vi "fpga_transmission_control_3V8.vi"() -> ()   [LabVIEW 2017]
uses:
  Control 1.ctl
  <vilib>/Platform/TimedLoop/XDataNode/timing_clust.ctl
  <vilib>/Platform/TimedLoop/XDataNode/nitl_modes.ctl
  <vilib>/Platform/TimedLoop/XDataNode/wakeup.ctl
  <vilib>/Instr/_visa.llb/VISA Configure Serial Port (Serial Instr).vi
  <vilib>/platform/TimedLoop/XDataNode/XDataNode.xnode
  <vilib>/Platform/TimedLoop/XDataNode/XDNodeRunTimeDep.lvlib
panel:
  out "Timer":dbl
  out "Output":bool
  out "outcome":u32
  out "currentType":string
  out "Time":dbl(slide) scale=0.0..100.0
  out "Progress":dbl(slide) scale=0.0..100.0
  in  "error in (no error)":errorcluster
  out "PWM":bool
  out "pattern":u32
  in  "Timeslot":bool
  out "type":string
  out "Kombi Chart":cluster{u16, i16}(graph)
  out "contingency":string
  in  "Array":T2(array[cluster]) {"duration" step=1}
  out "Timeslot":i32
  out "Sign":bool
  out "deleted portion":u8[](array[numeric])
  out "data":bool
  out "x-y":u16
  out "Error String":string
  out "error out":errorcluster
  out "Timing":u32
  out "Int_pixel":i16
  out "Pixel":u16(graph)
  out "AD_Value":i16
  in  "millisecond timer value 2":u32
  out "AD_Chart":i16(graph)
  in  "Path":path
  out "Read":bool
  in  "Stop Program":bool
  in  "Start":bool
  in  "VISA resource name":refnum<visa-resource-name>
  # "UR Elektronik Biologie\nTerminal V 3.8"
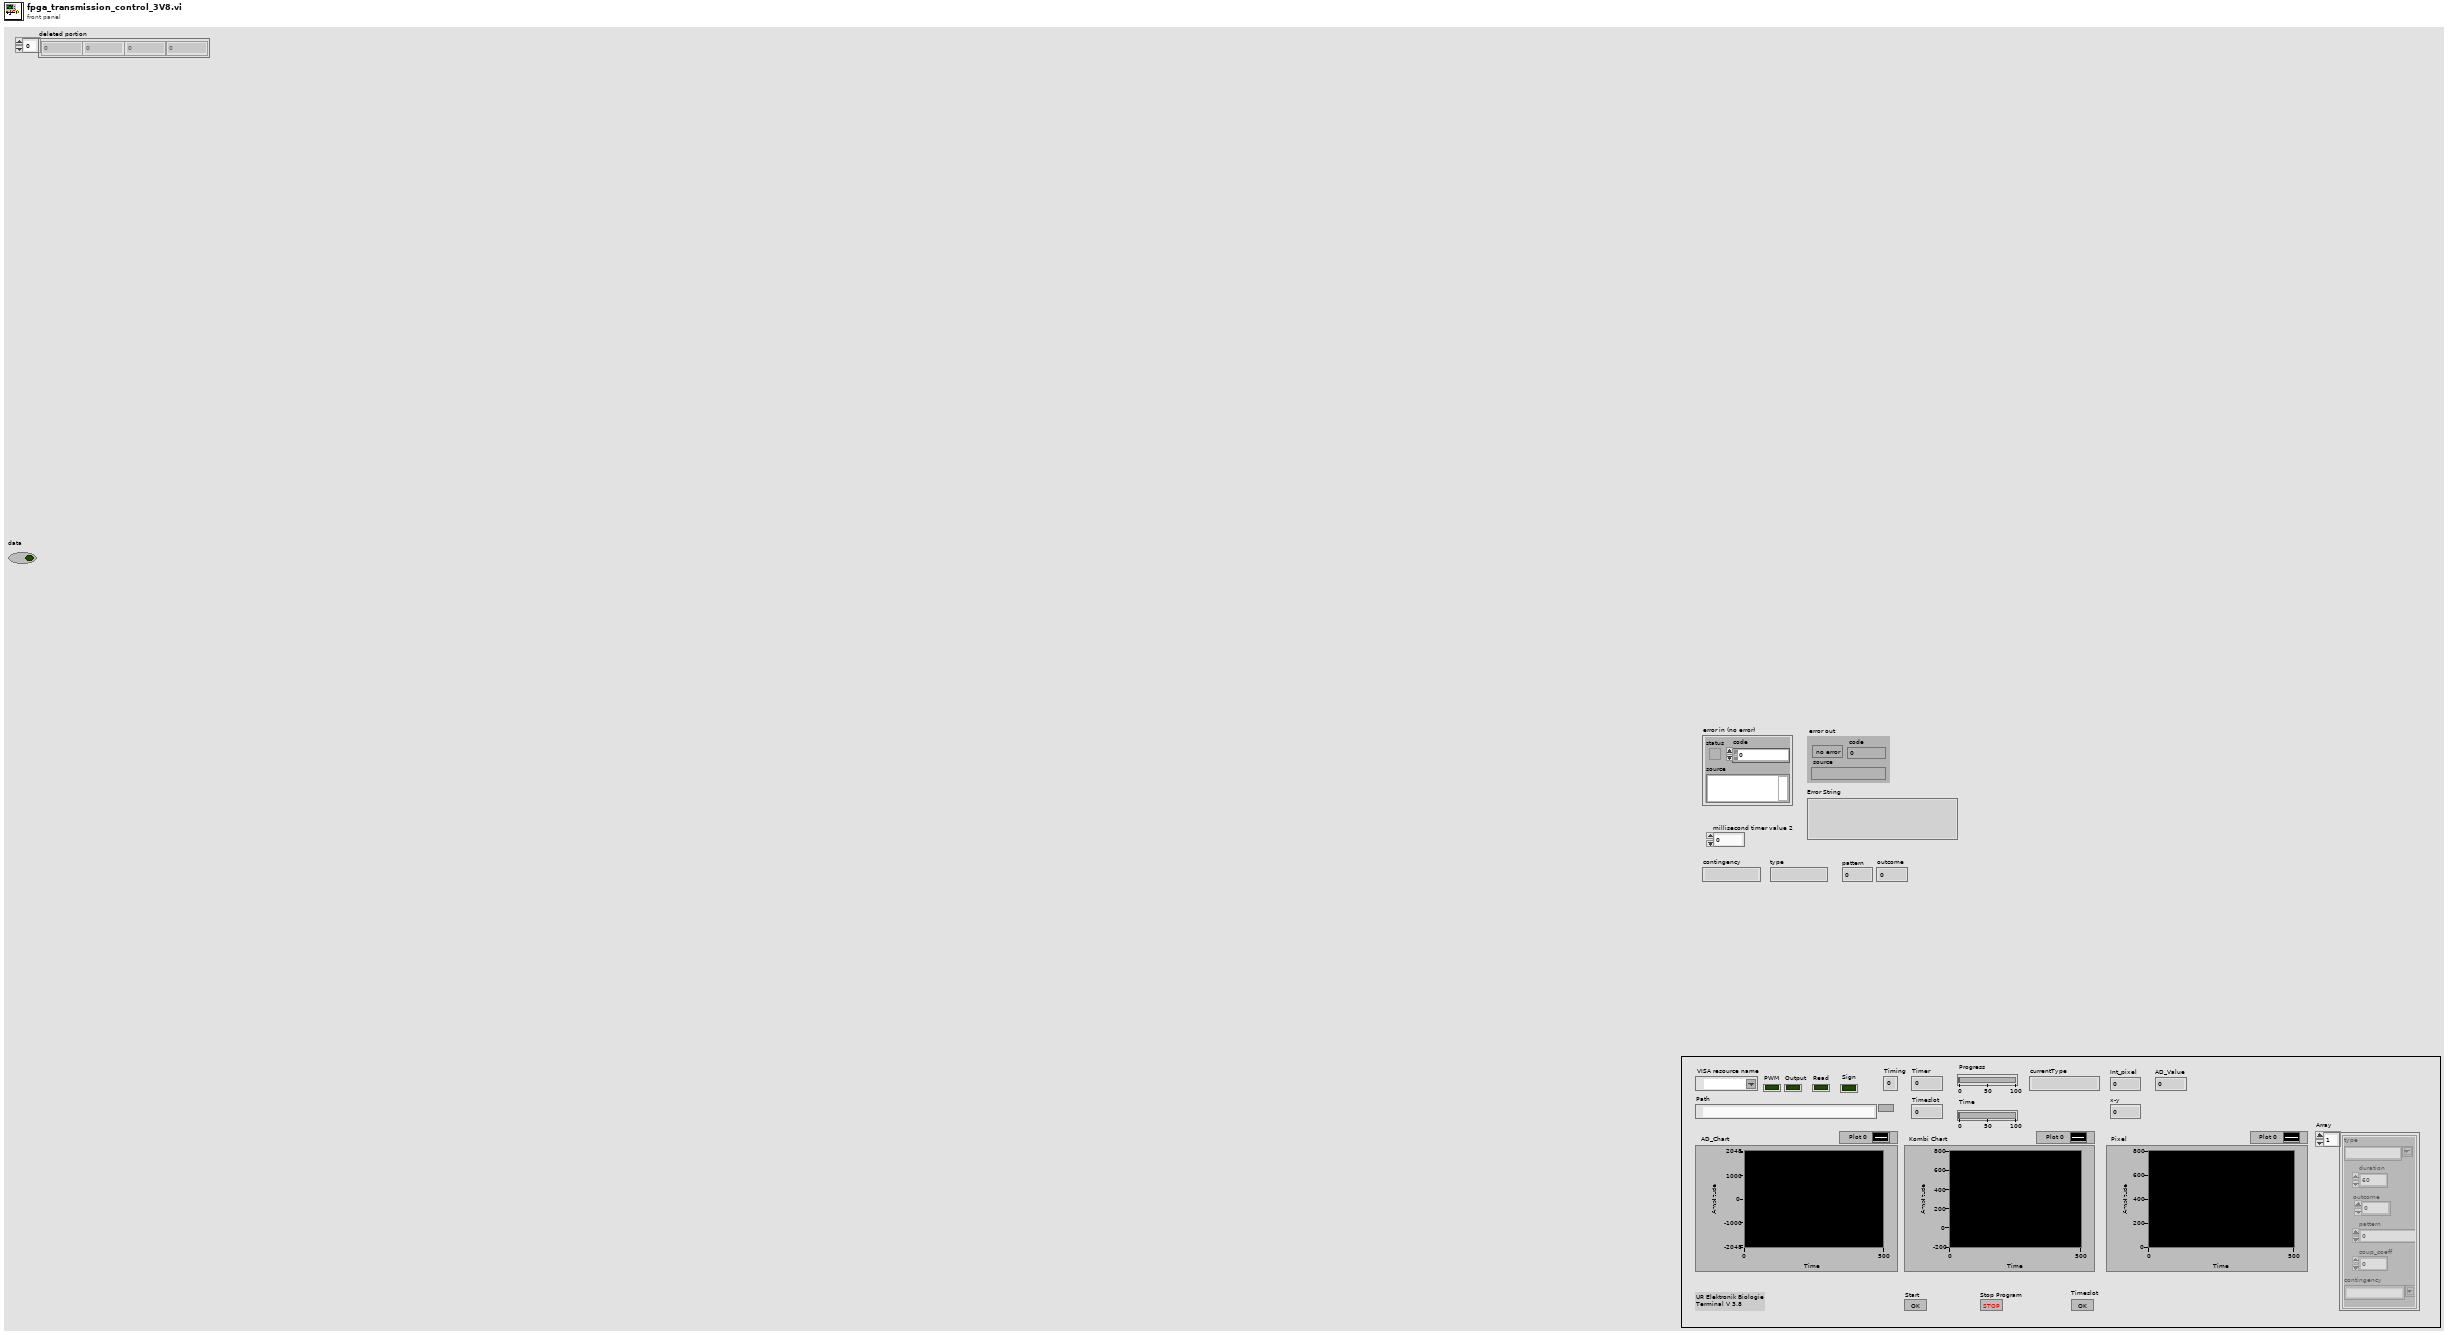
[diagram p1: front panel]
types:
  T1 = typedef "Control 1.ctl" = u32
  T2 = cluster{"type":string, "duration":T1, "outcome":u32, "pattern":u32, "coup_coeff":u32, "contingency":string}[]
  T3 = typedef "XDNodeRunTimeDep.lvlib/timing_clust.ctl" = cluster{"Expected End [f-1]":u64, "Actual End [f-1]":u64, "Finished Late? [f-1]":bool, "Expected End [i-1]":u64, "Actual End [i-1]":u64, "Finished Late? [i-1]":bool, "Expected Start [i]":u64, "Actual Start [i]":u64, "Expected Start [f]":u64, "Actual Start [f]":u64, "Source Name":string, "Structure Name":string, "Period":i64, "Deadline":i64, "Offset":i64, "Start":i64, "Priority":i32, "Timeout":i32, "Mode":T4, "Wakeup Reason":T5, "Error":errorcluster, "Source Type":string, "Secondary Source Type":string, "Global End Time":u64, "Global Start Time":u64, "Frame Duration":u64, "Iteration Duration":u64, "Assigned CPU":i32, "I/O Scan Engine Mode":u32}
  T4 = typedef "XDNodeRunTimeDep.lvlib/nitl_modes.ctl" = enum32{"No Change", "Process missed periods, maintain original phase", "Discard missed periods, maintain original phase", "Process missed periods, ignore original phase", "Discard missed periods, ignore original phase"}
  T5 = typedef "XDNodeRunTimeDep.lvlib/wakeup.ctl" = enum32{"Normal", "Aborted", "Asynchronous wakeup", "Timing source error", "Timed loop error", "Timeout"}
  T6 = cluster{"String":string, i32, i32, u32, u32, "String":string}[]
  T7 = enum16{"Idel", "State1", "State2", "State3", "State4"}
  T8 = enum16{"open", "replace", "create", "open or create", "replace or create", "replace or create with confirmation"}
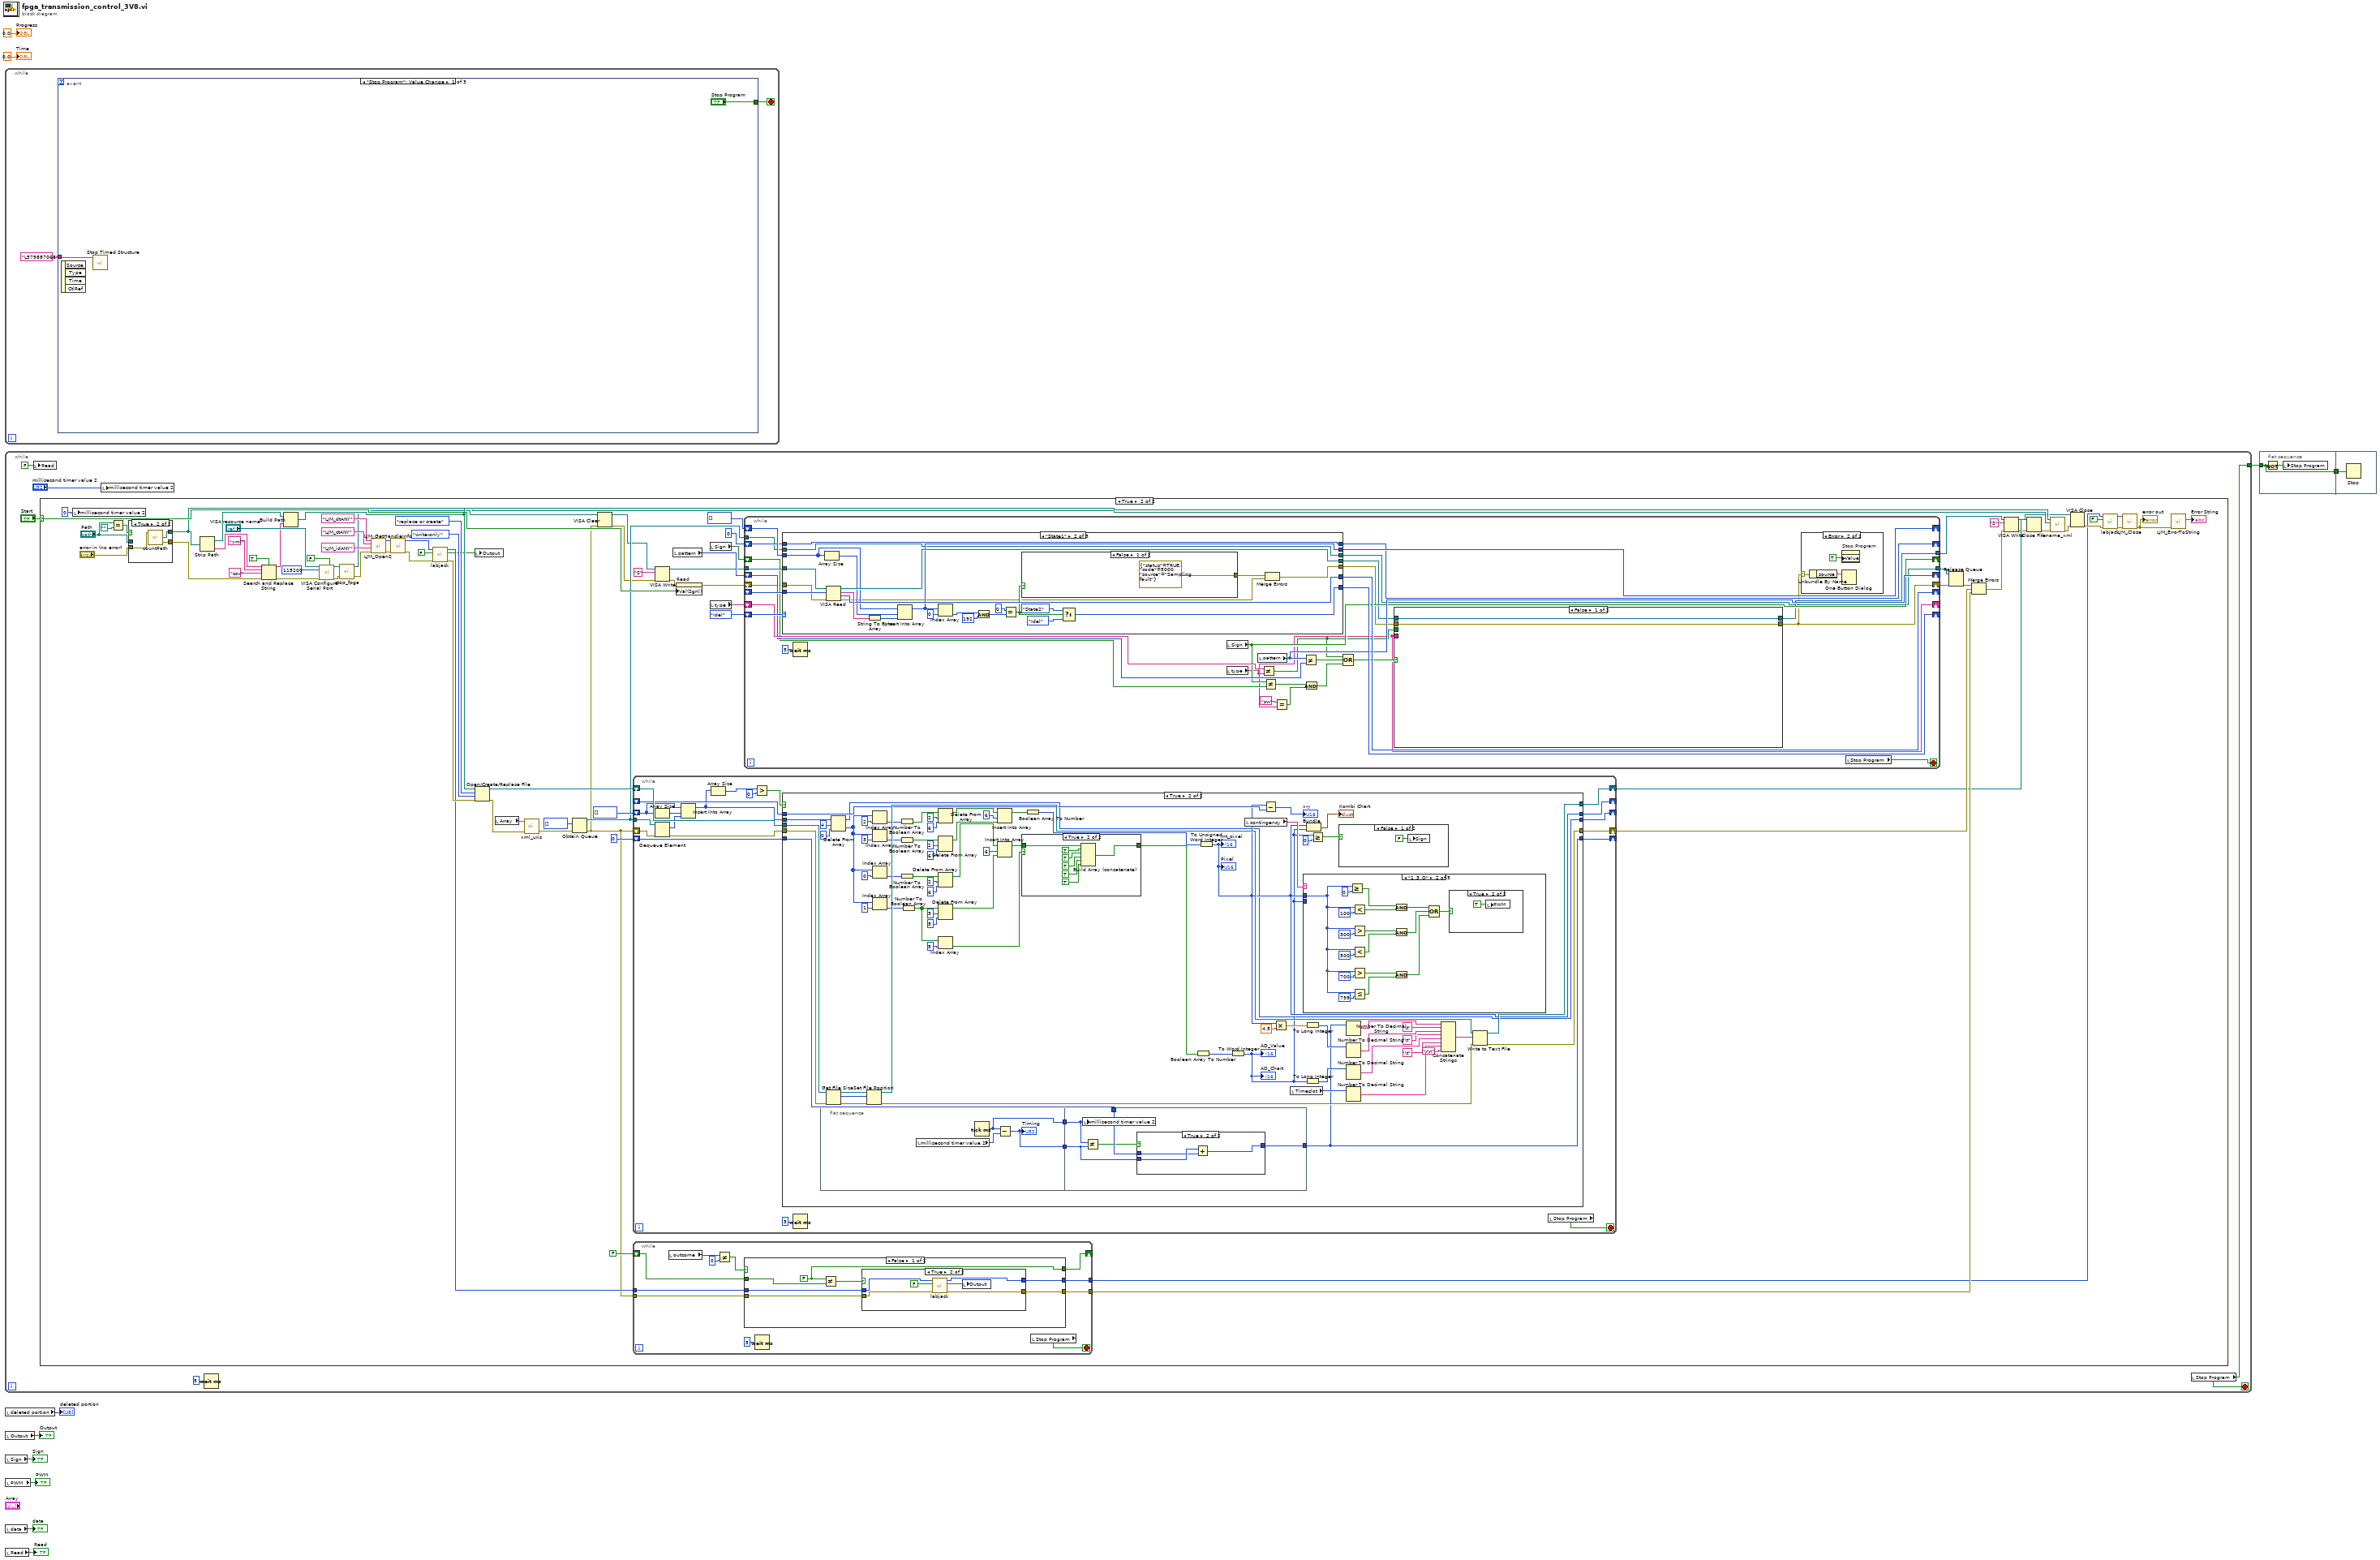
[diagram p0: block diagram]
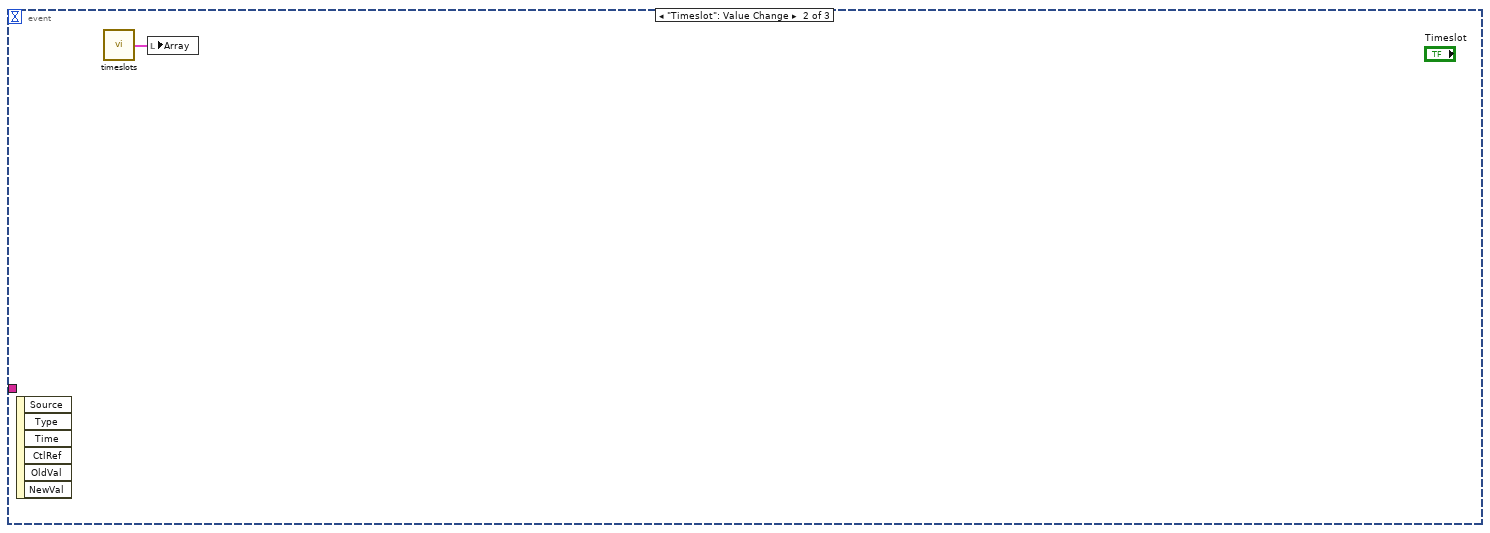
[diagram p2: hidden frame]
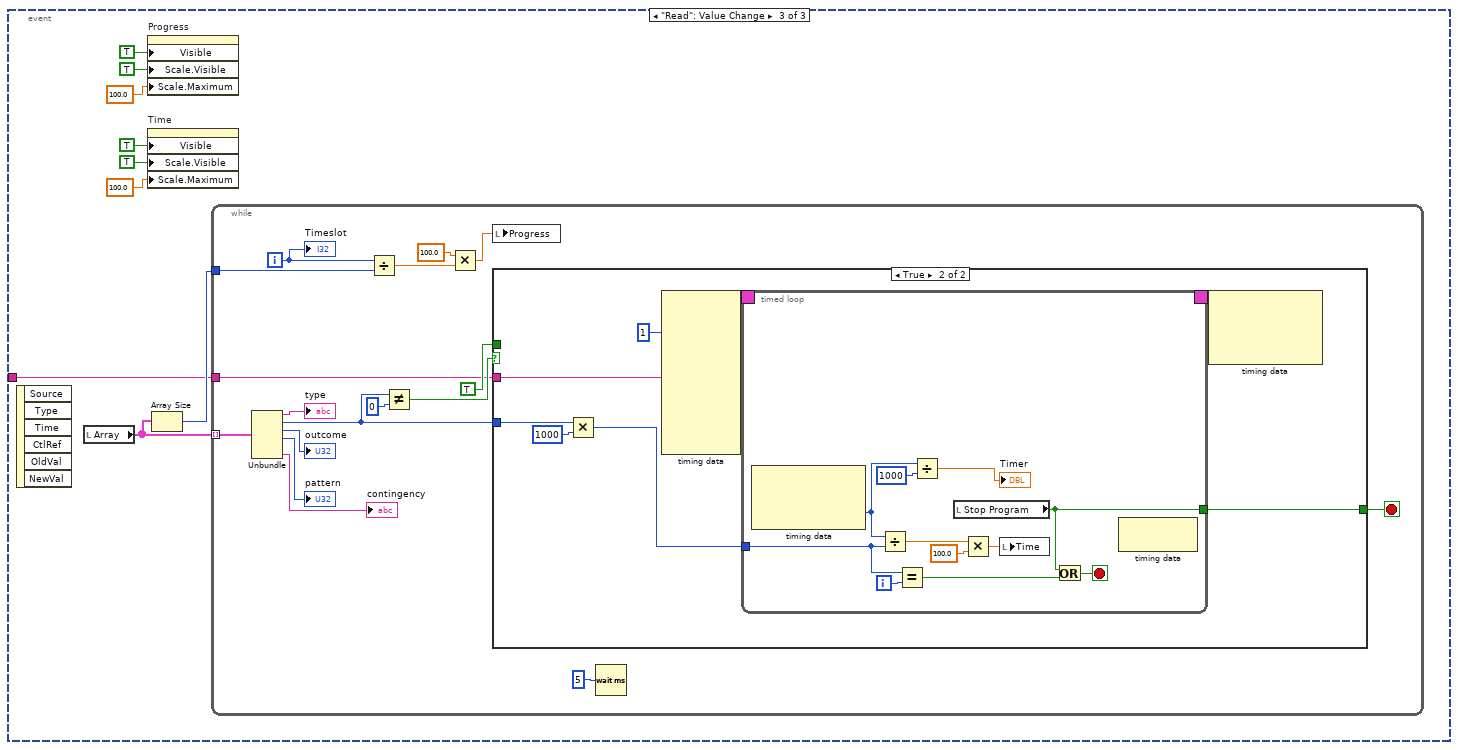
[diagram p3: hidden frame]
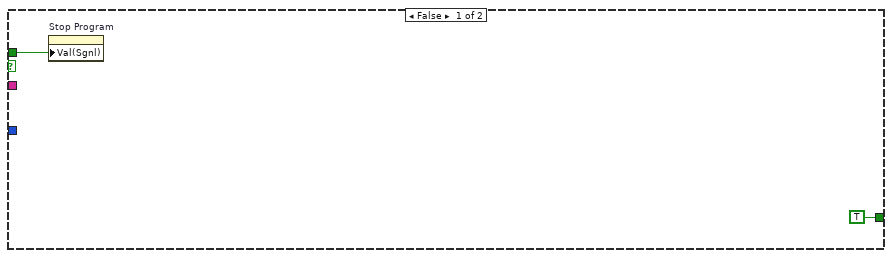
[diagram p4: hidden frame]
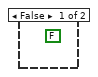
[diagram p5: hidden frame]
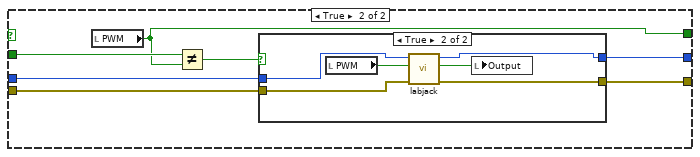
[diagram p8: hidden frame]
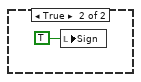
[diagram p11: hidden frame]
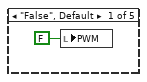
[diagram p12: hidden frame]
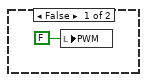
[diagram p13: hidden frame]
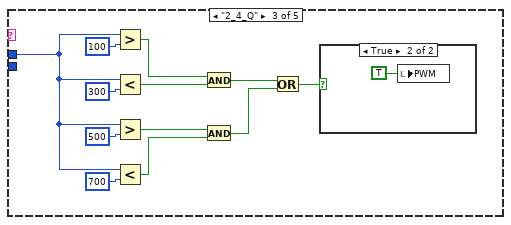
[diagram p14: hidden frame]
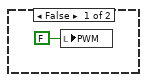
[diagram p15: hidden frame]
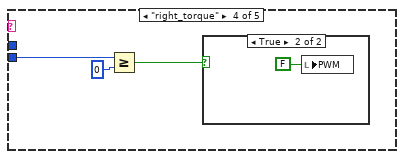
[diagram p16: hidden frame]
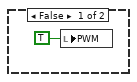
[diagram p17: hidden frame]
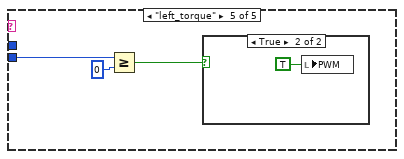
[diagram p18: hidden frame]
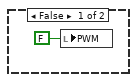
[diagram p19: hidden frame]
diagram:
  n1 = while {
    stop <- w12 stop-if-true
    n2 = event shown="[0] \"Stop Program\": Value Change" {
      selector: _ -> [_ _ _]
      dyn-events: _ -> [_ _ _]
      timeout: _ -> [_ _ _]
      tunnel: ["Stop Program" _ _] -> w12
      tunnel: "L579887068" ("Structure Name") -> [w13 _ w16]
      event "Stop Program": Value Change {
        n3 = event-data() -> ()  [unwired: 1 in, 4 out]
        n4 = call <vilib>:"Stop Timed Structure.vi"("name"=w13) -> ()  [unwired: 10 in, 1 out]
      }
      event "Timeslot": Value Change {
        n5 = event-data() -> ()  [unwired: 1 in, 6 out]
        n6 = call "timeslots.vi"() -> ("array of clusters"=w15:T6)  [unwired: 2 in]
        n7 = local write "Array"(w15) -> ()
      }
      event "Read": Value Change {
        n8 = event-data() -> ()  [unwired: 1 in, 6 out]
        n9 = local read "Array"() -> (w24:T2)
        n10 = property on="Progress" class="Slide (strict)"("Visible"=TRUE, "Scale.Visible"=TRUE ("Visible"), "Scale.Maximum"=100.0 ("Scale.Range:Maximum")) -> ()  [unwired: 2 in, 2 out]
        n11 = property on="Time" class="Slide (strict)"("Visible"=TRUE, "Scale.Visible"=TRUE ("Visible"), "Scale.Maximum"=100.0 ("Scale.Range:Maximum")) -> ()  [unwired: 2 in, 2 out]
        n12 = Array Size(array=w24) -> (size(s)=w23:i32)
        n13 = while {
          tunnel: w24 -> [w41] mode=indexing
          tunnel: w23 -> [w34]
          tunnel: w16 -> [w25]
          i -> [w33]
          stop <- w26 stop-if-true
          n14 = Unbundle(w41) -> ("type"=→"type":string, "duration"=w27:T1, "outcome"=→"outcome":u32, "pattern"=→"pattern":u32, "contingency"=→"contingency":string)  [unwired: 1 out]
          n15 = Divide(x=w33, y=w34) -> (x/y=w32:dbl)
          n16 = Not Equal?(x=w27, y=u32 0) -> (x != y?=w39:bool)
          n17 = Multiply(x=100.0 ("y"), y=w32) -> (x*y=w30:dbl)
          n18 = local write "Progress"(w30) -> ()
          n19 = case shown="True" w39 {
            tunnel: w27 -> [_ w48]
            tunnel: [TRUE w45] -> w26
            tunnel: TRUE -> [w42 _]
            tunnel: w25 -> [_ w44]
            frame False {
              n20 = property on="Stop Program" class="Bool (strict)"("Val(Sgnl)"=w42) -> ()  [unwired: 2 in, 2 out]
            }
            frame True {
              n21 = Multiply(x=w48, y=T1 1000) -> (x*y=w46:T1)
              n22 = node-c288(i64 1 ("Period"), w44) -> (w51:T3)  [unwired: 7 in]
              n23 = timed-loop {
                timing: w51 -> [_]
                timing-out: [_] -> w50
                tunnel: w46 -> [w58]
                tunnel: [w59] -> w45
                i -> [w62]
                stop <- w61 stop-if-true
                n24 = node-c288() -> (w54:i64)  [unwired: 1 in, 2 out]
                n25 = Divide(x=w54, y=w58) -> (x/y=w56:dbl)
                n26 = Equal?(x=w58, y=w62) -> (x = y?=w60:bool)
                n27 = Divide(x=w54, y=i64 1000) -> (x/y=→"Timer":dbl)
                n28 = local read "Stop Program"() -> (w59:bool)
                n29 = Multiply(x=w56, y=100.0) -> (x*y=w57:dbl)
                n30 = local write "Time"(w57) -> ()
                n31 = Or(x=w59, y=w60) -> (x .or. y?=w61:bool)
                n32 = node-c288() -> ()  [unwired: 1 in, 1 out]
              }
              n33 = node-c288(w50) -> ()  [unwired: 3 out]
            }
          }
          n34 = Wait (ms)(milliseconds to wait=u32 5) -> ()  [unwired: 1 out]
          "Timeslot" <- w33
        }
      }
    }
  }
  n35 = while {
    tunnel: [w74] -> w10
    stop <- w74 stop-if-true
    n36 = local write "Read"(FALSE) -> ()
    n37 = case shown="True" "Start" {
      selector: "Start" -> [_ w147]
      frame False {
        (unwired) FALSE
      }
      frame True {
        n38 = local write "millisecond timer value 2"(u32 0 ("millisecond timer value 2")) -> ()
        n39 = Equal?(x="Path", y=path "") -> (x = y?=w134:bool)
        n40 = case shown="True" w134 {
          tunnel: [w155 w158] -> w100
          tunnel: "Path" -> [w155 _]
          tunnel: [w154 w157] -> w109
          tunnel: "error in (no error)" -> [w154 w156]
          frame False {
          }
          frame True {
            n41 = call "countPath.vi"("error in (no error)"=w156) -> ("error out"=w157:errorcluster, "appended path"=w158:path)
          }
        }
        n42 = Strip Path(path=w100) -> (stripped path=w113:path, name=w112:string)
        n43 = Search and Replace String(case sensitive?=TRUE ("ignore case? (F)"), input string=w112, search string="xml", replace string="csv" ("replace string (\"\")"), error in=w109) -> (result string=w106:string, error out=w108:errorcluster)  [unwired: 3 in, 2 out]
        n44 = Build Path(base path=w113, name or relative path=w106) -> (appended path=w101:path)
        n45 = call-poly "VISA Configure Serial Port"("VISA resource name"="VISA resource name", "Enable Termination\nChar (T)"=FALSE ("Enable Termination\nChar (T)"), "baud rate (9600)"=u32 115200, "error in (no error)"=w108) -> ("VISA resource name out"=w92:refnum<visa-resource-name>, "error out"=w91:errorcluster)  [unwired: 10 in]
        n46 = call "stop_fpga.vi"("error in (no error)"=w91, "reference"=w92) -> ("error out"=w90:errorcluster, "VISA resource name out"=w80:refnum<visa-resource-name>)  [unwired: 2 in]
        n47 = call "LJM_OpenS.vi"("error in"=w90, "Identifier"="LJM_idANY", "ConnectionType"="LJM_ctANY", "DeviceType"="LJM_dtANY") -> ("error out"=w137:errorcluster, "Handle"=w136:i32)  [unwired: 6 in]
        n48 = call "LJM_GetHandleInfo.vi"("error in"=w137, "Handle In"=w136) -> ("error out"=w139:errorcluster, "Handle Out"=w138:i32)  [unwired: 2 in, 6 out]
        n49 = call "labjack.vi"("error out"=w139, "Boolean"=FALSE, "Handle Out"=w138) -> ("error out 2"=w142:errorcluster, "Boolean 2"=w99:bool, "Handle Out 2"=w141:i32)  [unwired: 6 in]
        n50 = local write "Output"(w99) -> ()
        n51 = Open/Create/Replace File(file path (use dialog)=w101, error in=w142, operation (0:open)=T8."replace or create", access (0:read/write)=enum16{"read/write", "read-only", "write-only"}."write-only") -> (refnum out=w116:refnum<file>, error out=w114:errorcluster)  [unwired: 2 in, 1 out]
        n52 = local read "Array"() -> (w115:T2)
        n53 = call "xml_uris.vi"("error in"=w114, "Array"=w115) -> ("error out"=w82:errorcluster)  [unwired: 2 in, 2 out]
        n54 = Obtain Queue(element data type=u8[] [], error in (no error)=w82) -> (queue out=w86:refnum<queue>, error out=w81:errorcluster)  [unwired: 3 in, 1 out]
        n55 = VISA Clear(VISA resource name=w80, error in (no error)=w81) -> (VISA resource name out=w79:refnum<visa-resource-name>, error out=w77:errorcluster)
        n56 = while {
          shift-right: [w218] -> w104
          shift-left: w116 -> [w219]
          shift-right: [w215] -> _
          shift-left: _ -> [w217]
          shift-right: [w214] -> w105
          shift-left: w81 -> [w201]
          shift-right: [w213] -> _
          shift-left: u32 0 -> [w212]
          shift-right: [w209] -> _
          shift-left: u8[] [] -> [w210]
          tunnel: w86 -> [w205]
          stop <- w216 stop-if-true
          n57 = Array Size(array=w210) -> (size(s)=w208:i32)
          n58 = Dequeue Element(queue=w205, error in (no error)=w201) -> (element=w204:u8[], error out=w200:errorcluster)  [unwired: 1 in, 2 out]
          n59 = Insert Into Array(array=w210, index=w208, new element=w204) -> (w203:u8[])
          n60 = Array Size(array=w203) -> (size(s)=w202:i32)
          n61 = Greater?(x=w202, y=0) -> (0:w206:bool)
          n62 = case shown="True" w206 {
            tunnel: w200 -> [w224 w248]
            tunnel: [w224 w292] -> w214
            tunnel: w219 -> [w223 w254]
            tunnel: [w223 w291] -> w218
            tunnel: [w222 w231] -> w215
            tunnel: w217 -> [w222 w249]
            tunnel: [w221 w235] -> w213
            tunnel: w212 -> [w221 w236]
            tunnel: w203 -> [w220 w229]
            tunnel: [w220 w225] -> w209
            frame False {
            }
            frame True {
              n63 = flat-sequence {
                tunnel: [w353] -> w290
                tunnel: [w352] -> w237
                tunnel: w290 -> [w356]
                tunnel: w237 -> [w357]
                tunnel: [w359] -> w235
                tunnel: w236 -> [w358]
                frame #0 {
                  n64 = local read "millisecond timer value 2"() -> (w354:u32)
                  n65 = Tick Count (ms)() -> (millisecond timer value=w353:u32)
                  n66 = Subtract(x=w353, y=w354) -> (x-y=w352:u32)
                  "Timing" <- w352
                }
                frame #1 {
                  n67 = local write "millisecond timer value 2"(w356) -> ()
                  n68 = Not Equal?(x=w356, y=w357) -> (x != y?=w355:bool)
                  n69 = case shown="True" w355 {
                    tunnel: w357 -> [_ w363]
                    tunnel: [u32 0 w362] -> w359
                    tunnel: w358 -> [_ w361]
                    frame False {
                    }
                    frame True {
                      n70 = Add(x=w363, y=w361) -> (x+y=w362:u32)
                    }
                  }
                }
              }
              n71 = Get File Size(file=w254, error in=w248) -> (refnum out=w297:refnum<file>, size (in bytes)=w296:i64, 0:w295:errorcluster)
              n72 = Delete From Array(array=w229, length=4, index=0) -> (deleted portion=w226:u8[], array with subset deleted=w225:u8[])
              n73 = Set File Position(offset (in bytes) (0)=w296, refnum=w297, error in=w295) -> (refnum out=w293:refnum<file>, error out=w294:errorcluster)  [unwired: 1 in]
              n74 = Index Array(array=w226, index=2) -> (element=w251:u8)
              n75 = Index Array(array=w226, index=3) -> (element=w250:u8)
              n76 = Index Array(array=w226, index=0) -> (element=w253:u8)
              n77 = Index Array(array=w226, index=1) -> (element=w252:u8)
              n78 = Number To Boolean Array(number=w251) -> (Boolean array=w272:bool[])
              n79 = Number To Boolean Array(number=w250) -> (Boolean array=w275:bool[])
              n80 = Number To Boolean Array(number=w253) -> (Boolean array=w262:bool[])
              n81 = Number To Boolean Array(number=w252) -> (Boolean array=w281:bool[])
              n82 = Delete From Array(array=w272, length=2, index=6 ("length")) -> (array with subset deleted=w285:bool[])  [unwired: 1 out]
              n83 = Delete From Array(array=w275, length=2, index=6) -> (array with subset deleted=w286:bool[])  [unwired: 1 out]
              n84 = Delete From Array(array=w262, length=2, index=6 ("length")) -> (array with subset deleted=w265:bool[])  [unwired: 1 out]
              n85 = Delete From Array(array=w281, length=3, index=5) -> (array with subset deleted=w270:bool[])  [unwired: 1 out]
              n86 = Index Array(array=w281, index=5) -> (element=w283:bool)
              n87 = Insert Into Array(array=w285, index=6, new element=w286) -> (w279:bool[])
              n88 = Insert Into Array(array=w265, index=6, new element=w270) -> (w267:bool[])
              n89 = case shown="True" w283 {
                tunnel: w267 -> [w344 w351]
                tunnel: [w344 w346] -> w284
                frame False {
                }
                frame True {
                  n90 = Build Array (concatenate)(w351, TRUE ("new element/subarray"), TRUE ("new element/subarray"), TRUE ("new element/subarray"), TRUE ("new element/subarray"), TRUE ("element")) -> (w346:bool[])
                }
              }
              n91 = Boolean Array To Number(Boolean array=w279) -> (number=w280:u32)
              n92 = Boolean Array To Number(Boolean array=w284) -> (number=w271:u32)
              n93 = To Unsigned Word Integer(number=w280) -> (unsigned 16bit integer=w231:u16)
              "Pixel" <- w231
              "Int_pixel" <- w231
              n94 = To Word Integer(number=w271) -> (16bit integer=w230:i16)
              "AD_Chart" <- w230
              "AD_Value" <- w230
              n95 = local read "contingency"() -> (w238:string)
              n96 = Subtract(x=w231, y=w249) -> (x-y=→"x-y":u16)
              n97 = Multiply(x=w231, y=4.5) -> (x*y=w240:dbl)
              n98 = local read "Timeslot"() -> (w244:i32)
              n99 = case shown="\"1_3_Q\"" w238 {
                tunnel: w231 -> [_ w302 w328 _ _]
                tunnel: w230 -> [_ _ _ w334 w339]
                frame "False", Default {
                  n100 = local write "PWM"(FALSE ("pwm")) -> ()
                }
                frame "1_3_Q" {
                  n101 = Greater Or Equal?(x=w302, y=u16 0 ("x")) -> (x >= y?=w301:bool)
                  n102 = Less?(x=w302, y=u16 100) -> (x < y?=w312:bool)
                  n103 = Greater?(x=w302, y=u16 300 ("a")) -> (0:w314:bool)
                  n104 = Less?(x=w302, y=u16 500 ("b")) -> (x < y?=w313:bool)
                  n105 = Greater?(x=w302, y=u16 700) -> (0:w311:bool)
                  n106 = Less Or Equal?(x=w302, y=u16 799) -> (x <= y?=w309:bool)
                  n107 = And(x=w301, y=w312) -> (x .and. y?=w307:bool)
                  n108 = And(x=w314, y=w313) -> (x .and. y?=w306:bool)
                  n109 = And(x=w311, y=w309) -> (x .and. y?=w305:bool)
                  n110 = Compound Arithmetic op=OR(w307, w306, w305) -> (w304:bool)
                  n111 = case shown="True" w304 {
                    frame False {
                      n112 = local write "PWM"(FALSE ("pwm")) -> ()
                    }
                    frame True {
                      n113 = local write "PWM"(TRUE ("pwm")) -> ()
                    }
                  }
                }
                frame "2_4_Q" {
                  n114 = Greater?(x=w328, y=u16 100 ("x")) -> (0:w323:bool)
                  n115 = Less?(x=w328, y=u16 300) -> (x < y?=w324:bool)
                  n116 = Greater?(x=w328, y=u16 500 ("a")) -> (0:w327:bool)
                  n117 = Less?(x=w328, y=u16 700 ("b")) -> (x < y?=w325:bool)
                  n118 = And(x=w323, y=w324) -> (x .and. y?=w322:bool)
                  n119 = And(x=w327, y=w325) -> (x .and. y?=w326:bool)
                  n120 = Or(x=w322, y=w326) -> (x .or. y?=w321:bool)
                  n121 = case shown="True" w321 {
                    frame False {
                      n122 = local write "PWM"(FALSE ("pwm")) -> ()
                    }
                    frame True {
                      n123 = local write "PWM"(TRUE ("pwm")) -> ()
                    }
                  }
                }
                frame "right_torque" {
                  n124 = Greater Or Equal?(x=w334, y=i16 0) -> (x >= y?=w335:bool)
                  n125 = case shown="True" w335 {
                    frame False {
                      n126 = local write "PWM"(TRUE ("pwm")) -> ()
                    }
                    frame True {
                      n127 = local write "PWM"(FALSE ("pwm")) -> ()
                    }
                  }
                }
                frame "left_torque" {
                  n128 = Greater Or Equal?(x=w339, y=i16 0) -> (x >= y?=w340:bool)
                  n129 = case shown="True" w340 {
                    frame False {
                      n130 = local write "PWM"(FALSE ("pwm")) -> ()
                    }
                    frame True {
                      n131 = local write "PWM"(TRUE ("pwm")) -> ()
                    }
                  }
                }
              }
              n132 = To Long Integer(number=w240) -> (32bit integer=w239:i32)
              n133 = To Long Integer(number=w230) -> (32bit integer=w242:i32)
              n134 = Bundle(w231, w230) -> (→"Kombi Chart":cluster{u16, i16})  [unwired: 1 in]
              n135 = Greater Or Equal?(x=w230, y=i16 0) -> (x >= y?=w232:bool)
              n136 = case shown="False" w232 {
                frame False {
                  n137 = local write "Sign"(FALSE) -> ()
                }
                frame True {
                  n138 = local write "Sign"(TRUE) -> ()
                }
              }
              n139 = Number To Decimal String(number=w235) -> (decimal integer string=w247:string)  [unwired: 1 in]
              n140 = Number To Decimal String(number=w239) -> (decimal integer string=w287:string)  [unwired: 1 in]
              n141 = Number To Decimal String(number=w242) -> (decimal integer string=w245:string)  [unwired: 1 in]
              n142 = Number To Decimal String(number=w244) -> (decimal integer string=w243:string)  [unwired: 1 in]
              n143 = Concatenate Strings(w247, "\t" ("string"), w287, "\t" ("string"), w245, "\t" ("string"), w243, "\r\n") -> (w255:string)
              n144 = Write to Text File(file (use dialog)=w293, text=w255, error in=w294) -> (refnum out=w291:refnum<file>, error out=w292:errorcluster)  [unwired: 1 in, 1 out]
            }
          }
          n145 = Wait (ms)(milliseconds to wait=u32 5) -> ()  [unwired: 1 out]
          n146 = local read "Stop Program"() -> (w216:bool)
        }
        n147 = while {
          tunnel: w141 -> [w167]
          tunnel: w81 -> [w166]
          shift-right: [w163] -> _
          shift-left: FALSE ("pwm") -> [w169]
          tunnel: [w165] -> w123
          tunnel: [w164] -> w148
          stop <- w168 stop-if-true
          n148 = local read "outcome"() -> (w162:u32)
          n149 = Not Equal?(x=w162, y=u32 0) -> (x != y?=w160:bool)
          n150 = case shown="False" w160 {
            tunnel: w169 -> [w172 w191]
            tunnel: w167 -> [w176 w186]
            tunnel: w166 -> [w174 w187]
            tunnel: [w175 w190] -> w165
            tunnel: [w173 w189] -> w164
            tunnel: [w171 w188] -> w163
            frame False {
              w171 = FALSE ("Boolean")
              n151 = Not Equal?(x=w171, y=w172) -> (x != y?=w170:bool)
              n152 = case shown="True" w170 {
                tunnel: w176 -> [w178 w184]
                tunnel: [w178 w183] -> w175
                tunnel: w174 -> [w177 w182]
                tunnel: [w177 w181] -> w173
                frame False {
                }
                frame True {
                  n153 = call "labjack.vi"("error out"=w182, "Boolean"=FALSE, "Handle Out"=w184) -> ("error out 2"=w181:errorcluster, "Boolean 2"=w179:bool, "Handle Out 2"=w183:i32)  [unwired: 6 in]
                  n154 = local write "Output"(w179) -> ()
                }
              }
            }
            frame True {
              n155 = local read "PWM"() -> (w188:bool)
              n156 = Not Equal?(x=w191, y=w188) -> (x != y?=w185:bool)
              n157 = case shown="True" w185 {
                tunnel: w186 -> [w193 w199]
                tunnel: w187 -> [w192 w198]
                tunnel: [w193 w197] -> w190
                tunnel: [w192 w196] -> w189
                frame False {
                }
                frame True {
                  n158 = local read "PWM"() -> (w195:bool)
                  n159 = call "labjack.vi"("error out"=w198, "Boolean"=w195, "Handle Out"=w199) -> ("error out 2"=w196:errorcluster, "Boolean 2"=w194:bool, "Handle Out 2"=w197:i32)  [unwired: 6 in]
                  n160 = local write "Output"(w194) -> ()
                }
              }
            }
          }
          n161 = Wait (ms)(milliseconds to wait=u32 5) -> ()  [unwired: 1 out]
          n162 = local read "Stop Program"() -> (w168:bool)
        }
        n163 = VISA Write(VISA resource name=w79, write buffer="S", error in (no error)=w77) -> (VISA resource name out=w78:refnum<visa-resource-name>, error out=w89:errorcluster)  [unwired: 1 out]
        n164 = local read "pattern"() -> (w119:u32)
        n165 = property on="Read" class="Bool (strict)"(error in=w89, "Val(Sgnl)"=w147) -> (error out=w76:errorcluster)  [unwired: 1 in, 1 out]
        n166 = local read "Sign"() -> (w118:bool)
        n167 = local read "type"() -> (w143:string)
        n168 = while {
          tunnel: w78 -> [w394]
          shift-right: [w388] -> _
          shift-left: u8[] [] -> [w393]
          tunnel: [w369] -> w95
          shift-right: [w392] -> _
          shift-left: T7."Idel" -> [w391]
          shift-right: [w390] -> _
          shift-left: _ -> [w389]
          shift-right: [w387] -> _
          shift-left: u8 0 -> [w386]
          shift-right: [w376] -> _
          shift-left: w143 -> [w384]
          shift-right: [w383] -> _
          shift-left: w119 -> [w382]
          shift-right: [w381] -> _
          shift-left: w118 -> [w380]
          tunnel: w86 -> [w368]
          tunnel: [w367] -> w83
          shift-right: [w364] -> w85
          shift-left: w76 -> [w365]
          stop <- w385 stop-if-true
          n169 = case shown="\"State1\"" w391 {
            tunnel: w394 -> [w512 w537 w557]
            tunnel: w365 -> [w513 w538 w551]
            tunnel: w393 -> [w516 w540 w564]
            tunnel: [w520 w542 w557] -> w370
            tunnel: [w519 w526 w550] -> w371
            tunnel: [w521 w539 w560] -> w392
            tunnel: [w518 w543 w558] -> w390
            tunnel: w389 -> [_ w544 w558]
            tunnel: [w516 w536 w563] -> w388
            tunnel: [w515 w535 u8 0] -> w387
            tunnel: w386 -> [w515 w535 _]
            tunnel: w368 -> [w510 w529 w553]
            tunnel: [w510 w529 w552] -> w367
            frame "Idel", Default {
              n170 = local write "data"(FALSE ("data")) -> ()
              n171 = property class="Serial Instr"(reference=w512, error in=w513) -> (reference out=w520:refnum<visa-resource-name>, error out=w519:errorcluster, "Serial Settings:Number of Bytes at Serial Port"=w518:u32)
              n172 = Greater Or Equal?(x=w518, y=u8 4) -> (x >= y?=w511:bool)
              n173 = Select(t=T7."State1", s=w511, f=T7."Idel") -> (s? t:f=w521:T7)
            }
            frame "State1" {
              n174 = Array Size(array=w540) -> (size(s)=w528:i32)
              n175 = VISA Read(VISA resource name=w537, byte count=w544, error in (no error)=w538) -> (VISA resource name out=w542:refnum<visa-resource-name>, read buffer=w545:string, return count=w543:u32, error out=w524:errorcluster)
              n176 = String To Byte Array(string=w545) -> (unsigned byte array=w541:u8[])
              n177 = Insert Into Array(array=w540, index=w528, new element=w541) -> (w536:u8[])
              n178 = Index Array(array=w536, index=0) -> (element=w533:u8)
              n179 = And(x=w533, y=u8 192) -> (x .and. y?=w532:u8)
              n180 = Equal?(x=u8 0, y=w532) -> (x = y?=w525:bool)
              n181 = case shown="False" w525 {
                tunnel: [errorcluster {"status"=TRUE, "code"=5000, "source"="Sampling fault"} ("error constant") errorcluster {"status"=FALSE, "code"=0, "source"=""} ("error constant")] -> w527
                frame False {
                }
                frame True {
                }
              }
              n182 = Select(t=T7."State2", s=w525, f=T7."Idel") -> (s? t:f=w539:T7)
              n183 = Merge Errors(w527, w524) -> (w526:errorcluster)
            }
            frame "State2" {
              n184 = Delete From Array(array=w564, length=4, index=0) -> (deleted portion=w554:u8[], array with subset deleted=w563:u8[])
              n185 = Array Size(array=w563) -> (size(s)=w562:i32)
              n186 = Enqueue Element(queue=w553, element=w554, error in (no error)=w551) -> (queue out=w552:refnum<queue>, error out=w550:errorcluster)  [unwired: 1 in, 1 out]
              n187 = Greater Or Equal?(x=w562, y=4) -> (x >= y?=w555:bool)
              n188 = Select(t=T7."State2", s=w555, f=T7."Idel") -> (s? t:f=w560:T7)
            }
          }
          n189 = Wait (ms)(milliseconds to wait=u32 5) -> ()  [unwired: 1 out]
          n190 = local read "Sign"() -> (w381:bool)
          n191 = local read "type"() -> (w376:string)
          n192 = local read "pattern"() -> (w383:u32)
          n193 = Not Equal?(x=w384, y=w376) -> (x != y?=w377:bool)
          n194 = Not Equal?(x=w381, y=w380) -> (x != y?=w373:bool)
          n195 = Equal?(x="sw", y=w376) -> (x = y?=w374:bool)
          n196 = Not Equal?(x=w383, y=w382) -> (x != y?=w379:bool)
          n197 = And(x=w373, y=w374) -> (x .and. y?=w372:bool)
          n198 = Compound Arithmetic op=OR(w377, w379, w372) -> (w378:bool)
          n199 = case shown="False" w378 {
            tunnel: w370 -> [w399 w403]
            tunnel: [w399 w406] -> w369
            tunnel: w371 -> [w398 w402]
            tunnel: [w398 w407] -> w364
            tunnel: w376 -> [_ w400]
            tunnel: w377 -> [_ w401]
            frame False {
            }
            frame True {
              n200 = case shown="True" w401 {
                tunnel: [w409 w415] -> w405
                tunnel: [w410 w414] -> w404
                tunnel: w403 -> [w410 w412]
                tunnel: w402 -> [w409 w411]
                frame False {
                }
                frame True {
                  n201 = VISA Write(VISA resource name=w412, write buffer="1W", error in (no error)=w411) -> (VISA resource name out=w414:refnum<visa-resource-name>, error out=w415:errorcluster)  [unwired: 1 out]
                }
              }
              n202 = case shown="\"fs\"" w400 {
                tunnel: w404 -> [w417 w424 w429 w437 w448 w485]
                tunnel: [w419 w423 w428 w431 w447 w484] -> w406
                tunnel: w405 -> [w416 w422 w427 w436 w450 w487]
                tunnel: [w418 w421 w426 w432 w449 w486] -> w408
                frame "False", Default {
                  n203 = VISA Write(VISA resource name=w417, write buffer="s4s", error in (no error)=w416) -> (VISA resource name out=w419:refnum<visa-resource-name>, error out=w418:errorcluster)  [unwired: 1 out]
                }
                frame "optomotorR" {
                  n204 = VISA Write(VISA resource name=w424, write buffer="s3r", error in (no error)=w422) -> (VISA resource name out=w423:refnum<visa-resource-name>, error out=w421:errorcluster)  [unwired: 1 out]
                }
                frame "optomotorL" {
                  n205 = VISA Write(VISA resource name=w429, write buffer="s3l", error in (no error)=w427) -> (VISA resource name out=w428:refnum<visa-resource-name>, error out=w426:errorcluster)  [unwired: 1 out]
                }
                frame "yt" {
                  n206 = local read "pattern"() -> (w435:u32)
                  n207 = VISA Write(VISA resource name=w437, write buffer="s1s", error in (no error)=w436) -> (VISA resource name out=w434:refnum<visa-resource-name>, error out=w433:errorcluster)  [unwired: 1 out]
                  n208 = case shown="9" w435 {
                    tunnel: w434 -> [w440 w444]
                    tunnel: w433 -> [w439 w443]
                    tunnel: [w439 w442] -> w432
                    tunnel: [w440 w441] -> w431
                    frame 0, Default {
                    }
                    frame 9 {
                      n209 = VISA Write(VISA resource name=w444, write buffer="D", error in (no error)=w443) -> (VISA resource name out=w441:refnum<visa-resource-name>, error out=w442:errorcluster)  [unwired: 1 out]
                    }
                  }
                }
                frame "sw" {
                  n210 = local read "pattern"() -> (w446:u32)
                  n211 = case shown="7" w446 {
                    tunnel: w450 -> [w451 w456 w472]
                    tunnel: [w451 w454 w471] -> w449
                    tunnel: w448 -> [w452 w457 w470]
                    tunnel: [w452 w455 w469] -> w447
                    frame 0, Default {
                    }
                    frame 8 {
                      n212 = local read "Sign"() -> (w453:bool)
                      n213 = case shown="False" w453 {
                        tunnel: w456 -> [w459 w466]
                        tunnel: [w458 w465] -> w454
                        tunnel: w457 -> [w461 w464]
                        tunnel: [w460 w463] -> w455
                        frame True {
                          n214 = VISA Write(VISA resource name=w461, write buffer="G", error in (no error)=w459) -> (VISA resource name out=w460:refnum<visa-resource-name>, error out=w458:errorcluster)  [unwired: 1 out]
                        }
                        frame False {
                          n215 = VISA Write(VISA resource name=w464, write buffer="B", error in (no error)=w466) -> (VISA resource name out=w463:refnum<visa-resource-name>, error out=w465:errorcluster)  [unwired: 1 out]
                        }
                      }
                    }
                    frame 7 {
                      n216 = local read "Sign"() -> (w468:bool)
                      n217 = case shown="True" w468 {
                        tunnel: w472 -> [w474 w481]
                        tunnel: [w473 w480] -> w471
                        tunnel: w470 -> [w476 w479]
                        tunnel: [w475 w478] -> w469
                        frame False {
                          n218 = VISA Write(VISA resource name=w476, write buffer="G", error in (no error)=w474) -> (VISA resource name out=w475:refnum<visa-resource-name>, error out=w473:errorcluster)  [unwired: 1 out]
                        }
                        frame True {
                          n219 = VISA Write(VISA resource name=w479, write buffer="B", error in (no error)=w481) -> (VISA resource name out=w478:refnum<visa-resource-name>, error out=w480:errorcluster)  [unwired: 1 out]
                        }
                      }
                    }
                  }
                }
                frame "fs" {
                  n220 = local read "pattern"() -> (w483:u32)
                  n221 = case shown="4" w483 {
                    tunnel: w487 -> [w488 w494 w499 w504 w509]
                    tunnel: [w488 w492 w497 w502 w507] -> w486
                    tunnel: w485 -> [w489 w493 w498 w503 w508]
                    tunnel: [w489 w491 w496 w501 w506] -> w484
                    frame 0, Default {
                    }
                    frame 3 {
                      n222 = VISA Write(VISA resource name=w493, write buffer="s3s", error in (no error)=w494) -> (VISA resource name out=w491:refnum<visa-resource-name>, error out=w492:errorcluster)  [unwired: 1 out]
                    }
                    frame 2 {
                      n223 = VISA Write(VISA resource name=w498, write buffer="s2s", error in (no error)=w499) -> (VISA resource name out=w496:refnum<visa-resource-name>, error out=w497:errorcluster)  [unwired: 1 out]
                    }
                    frame 1 {
                      n224 = VISA Write(VISA resource name=w503, write buffer="s1s", error in (no error)=w504) -> (VISA resource name out=w501:refnum<visa-resource-name>, error out=w502:errorcluster)  [unwired: 1 out]
                    }
                    frame 4 {
                      n225 = VISA Write(VISA resource name=w508, write buffer="s4s", error in (no error)=w509) -> (VISA resource name out=w506:refnum<visa-resource-name>, error out=w507:errorcluster)  [unwired: 1 out]
                    }
                  }
                }
              }
              n226 = feedback #1() -> (w407:errorcluster)  [unwired: 1 in]
              n227 = feedback-in #1(w408) -> ()
              "currentType" <- w400
            }
          }
          n228 = case shown="Error" w364 {
            selector: w364 -> [_ w396]
            frame No Error {
            }
            frame Error {
              n229 = Unbundle By Name(w396) -> ("source"=w395:string)
              n230 = property on="Stop Program" class="Bool (strict)"("Value"=TRUE) -> ()  [unwired: 2 in, 2 out]
              n231 = One Button Dialog(message=w395) -> ()  [unwired: 1 in, 1 out]
            }
          }
          n232 = local read "Stop Program"() -> (w385:bool)
        }
        n233 = Release Queue(queue=w83, error in (no error)=w85) -> (error out=w84:errorcluster)  [unwired: 1 in, 2 out]
        n234 = Merge Errors(w84, w105, w148) -> (w97:errorcluster)
        n235 = VISA Write(VISA resource name=w95, write buffer="S", error in (no error)=w97) -> (VISA resource name out=w94:refnum<visa-resource-name>, error out=w96:errorcluster)  [unwired: 1 out]
        n236 = Close File(refnum=w104, error in=w96) -> (error out=w103:errorcluster)  [unwired: 1 out]
        n237 = call "rename_xml.vi"("error in"=w103, "xml"=w100, "csv"=w101) -> ("error out"=w102:errorcluster)  [unwired: 4 in]
        n238 = VISA Close(VISA resource name=w94, error in (no error)=w102) -> (error out=w128:errorcluster)
        n239 = call "labjack.vi"("error out"=w128, "Boolean"=FALSE, "Handle Out"=w123) -> ("error out 2"=w129:errorcluster, "Handle Out 2"=w127:i32)  [unwired: 6 in, 1 out]
        n240 = call "LJM_Close.vi"("error in"=w129, "Handle"=w127) -> ("error out"=w126:errorcluster)  [unwired: 9 in]
        "error out" <- w126
        n241 = call "LJM_ErrorToString.vi"("error in"=w126) -> ("String"=→"Error String":string)  [unwired: 10 in]
      }
    }
    n242 = local write "millisecond timer value 2"("millisecond timer value 2") -> ()
    n243 = Wait (ms)(milliseconds to wait=u32 5) -> ()  [unwired: 1 out]
    n244 = local read "Stop Program"() -> (w74:bool)
  }
  n245 = local read "deleted portion"() -> (→"deleted portion":u8[])
  n246 = local read "Output"() -> (→"Output":bool)
  n247 = local read "Sign"() -> (→"Sign":bool)
  n248 = local read "PWM"() -> (→"PWM":bool)
  n249 = local read "data"() -> (→"data":bool)
  n250 = local read "Read"() -> (→"Read":bool)
  n251 = flat-sequence {
    tunnel: w10 -> [w569]
    tunnel: [w569] -> w9
    tunnel: w9 -> [w570]
    frame #0 {
      n252 = Not(x=w569) -> (.not. x?=w568:bool)
      n253 = local write "Stop Program"(w568) -> ()
    }
    frame #1 {
      n254 = Stop(stop? (T)=w570) -> ()
    }
  }
  "Progress" <- 0.0 ("Slide")
  "Time" <- 0.0 ("Progress 2")
